vi "4.vi"() -> ()   [LabVIEW 2017]
uses:
  <vilib>/measure/NI_MABase.lvlib
panel:
  out "大小":i32
  out "最小值":dbl
  out "dt":dbl
  out "Y":dbl[](array[numeric])
  out "波形图":waveform(dbl)(graph)
  in  "phase":dbl caption="相位" format="%.2p"
  in  "amplitude":dbl=1.0 caption="幅值" format="%.2p"
  in  "frequency":dbl=10.0 caption="频率" format="%.2p"
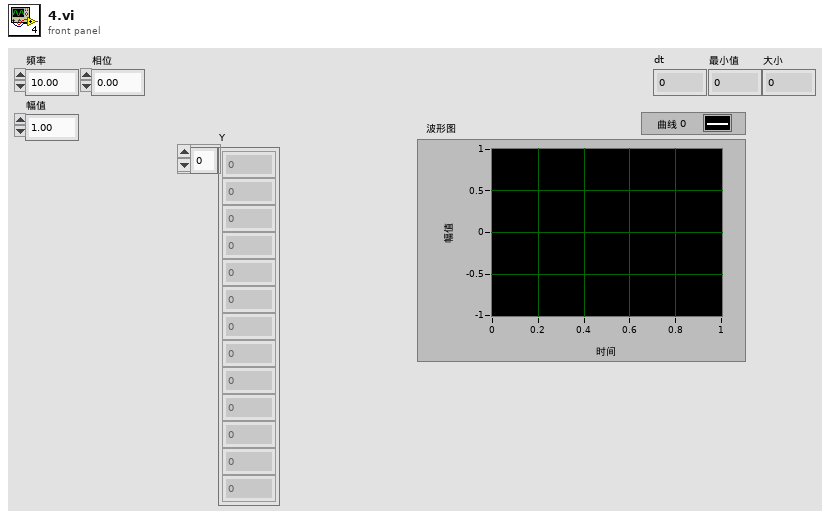
[diagram p1: front panel]
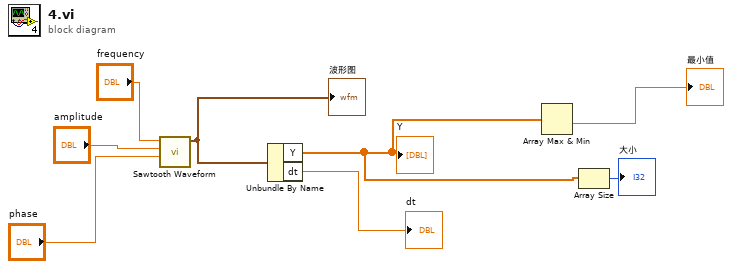
[diagram p0: block diagram]
diagram:
  n1 = call <vilib>:"Sawtooth Waveform.vi"("phase"="phase", "amplitude"="amplitude", "frequency"="frequency") -> ("signal out"=w4:waveform(dbl))  [unwired: 7 in, 1 out]
  "波形图" <- w4
  n2 = Unbundle By Name(w4) -> ("Y"=w2:dbl[], "dt"=→"dt":dbl)
  "Y" <- w2
  n3 = Array Max & Min(array=w2) -> (min value=→"最小值":dbl)  [unwired: 3 out]
  n4 = Array Size(array=w2) -> (size(s)=→"大小":i32)
